vi "ex_InitTreeControl.vi"(4 "error in (no error)":errorcluster, 5 "File refnum in":refnum<k20>, 7 "reference":refnum<vi>) -> (0 "error out":errorcluster)   [LabVIEW 2017]
doc: "Initializes a Tree Control with the contents of the input file"
uses:
  <vilib>/Platform/storage/Storage.llb/Get Property (String).vi
  <vilib>/Platform/storage/Storage.llb/Get Property (Storage Refnums).vi
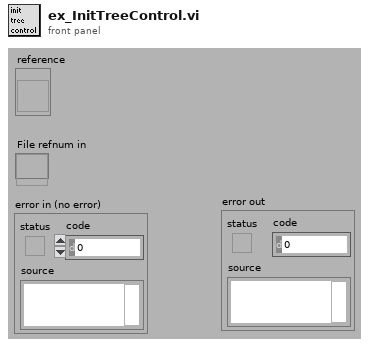
[diagram p1: front panel]
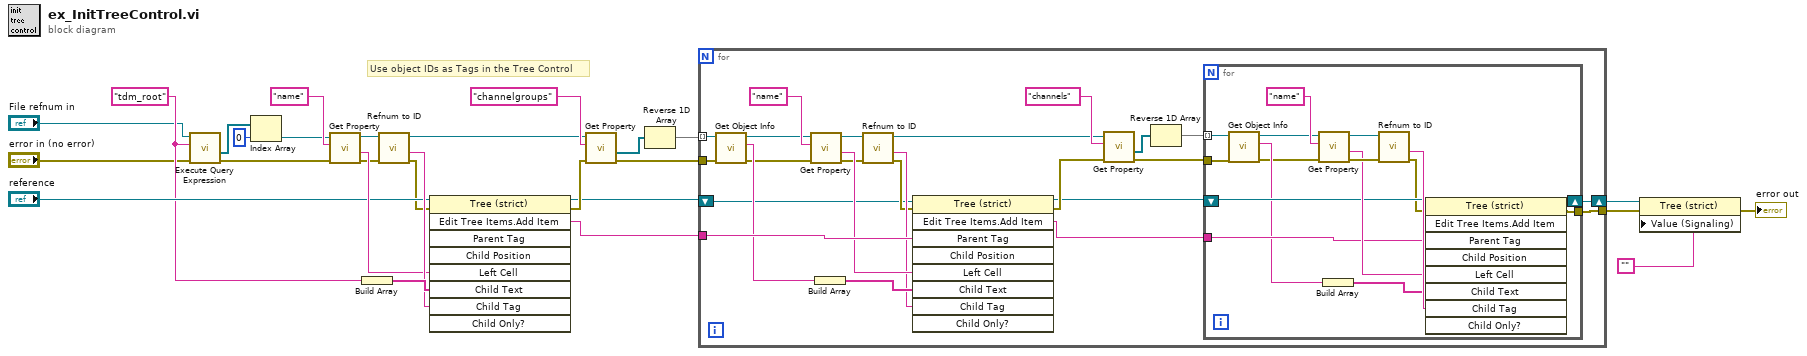
[diagram p0: block diagram]
diagram:
  w14 = "tdm_root" ("File")
  # "Use object IDs as Tags in the Tree Control"
  n1 = call <vilib>:"Execute Query Expression.vi"("error in (no error)"="error in (no error)", "object type"=w14, "storage refnum"="File refnum in") -> ("error out"=w16:errorcluster, "storage refnums"=w18:refnum<k20>[])  [unwired: 1 in, 2 out]
  n2 = Index Array(array=w18, index=0) -> (element=w19:refnum<k20>)
  n3 = call-poly <vilib>:"Get Property.vi"("error in (no error)"=w16, "Property name"="name" ("Name"), "storage refnum"=w19) -> ("error out"=w22:errorcluster, "Value"=w23:string, "storage refnum out"=w11:refnum<k20>)  [unwired: 6 out]
  n4 = Build Array(w14) -> (w25:string[])
  n5 = call <vilib>:"Refnum to ID.vi"("error in (no error)"=w22, "storage refnum"=w11) -> ("error out"=w10:errorcluster, "object ID"=w24:string, "storage refnum out"=w8:refnum<k20>)  [unwired: 3 out]
  n6 = invoke on="Invoke Node" class="Tree (strict)" method="Edit Tree Items.Add Item"(reference="reference", error in=w10, "Left Cell"=w23, "Child Text"=w25, "Child Tag"=w24) -> (reference out=w7:refnum<vi>, error out=w9:errorcluster, "Edit Tree Items:Add Item"=w27:string)  [unwired: 4 in, 6 out]
  n7 = call-poly <vilib>:"Get Property.vi"("error in (no error)"=w9, "Property name"="channelgroups" ("Channel groups"), "storage refnum"=w8) -> ("error out"=w26:errorcluster, "Value"=w1:refnum<k20>[])  [unwired: 7 out]
  n8 = Reverse 1D Array(array=w1) -> (reversed array=w2:refnum<k20>[])
  n9 = for {
    tunnel: w2 -> [w41] mode=indexing
    tunnel: w26 -> [w40]
    tunnel: w27 -> [w50]
    tunnel: [w42] -> w4
    shift-right: [w31] -> w6
    shift-left: w7 -> [w30]
    n10 = call <vilib>:"Get Object Info.vi"("error in (no error)"=w40, "storage refnum"=w41) -> ("error out"=w38:errorcluster, "object type"=w39:string, "storage refnum out"=w37:refnum<k20>)  [unwired: 7 out]
    n11 = call-poly <vilib>:"Get Property.vi"("error in (no error)"=w38, "Property name"="name" ("Name"), "storage refnum"=w37) -> ("error out"=w47:errorcluster, "Value"=w49:string, "storage refnum out"=w36:refnum<k20>)  [unwired: 6 out]
    n12 = Build Array(w39) -> (w48:string[])
    n13 = call <vilib>:"Refnum to ID.vi"("error in (no error)"=w47, "storage refnum"=w36) -> ("error out"=w34:errorcluster, "object ID"=w46:string, "storage refnum out"=w35:refnum<k20>)  [unwired: 3 out]
    n14 = invoke on="Invoke Node" class="Tree (strict)" method="Edit Tree Items.Add Item"(reference=w30, error in=w34, "Parent Tag"=w50, "Left Cell"=w49, "Child Text"=w48, "Child Tag"=w46) -> (reference out=w32:refnum<vi>, error out=w33:errorcluster, "Edit Tree Items:Add Item"=w45:string)  [unwired: 3 in, 6 out]
    n15 = call-poly <vilib>:"Get Property.vi"("error in (no error)"=w33, "Property name"="channels" ("Channels"), "storage refnum"=w35) -> ("error out"=w43:errorcluster, "Value"=w29:refnum<k20>[])  [unwired: 7 out]
    n16 = Reverse 1D Array(array=w29) -> (reversed array=w28:refnum<k20>[])
    n17 = for {
      tunnel: w43 -> [w57]
      tunnel: w45 -> [w61]
      tunnel: [w58] -> w42
      shift-right: [w53] -> w31
      shift-left: w32 -> [w60]
      tunnel: w28 -> [w52] mode=indexing
      n18 = call <vilib>:"Get Object Info.vi"("error in (no error)"=w57, "storage refnum"=w52) -> ("error out"=w54:errorcluster, "object type"=w56:string, "storage refnum out"=w55:refnum<k20>)  [unwired: 7 out]
      n19 = call-poly <vilib>:"Get Property.vi"("error in (no error)"=w54, "Property name"="name" ("Name"), "storage refnum"=w55) -> ("error out"=w65:errorcluster, "Value"=w63:string, "storage refnum out"=w66:refnum<k20>)  [unwired: 6 out]
      n20 = Build Array(w56) -> (w64:string[])
      n21 = call <vilib>:"Refnum to ID.vi"("error in (no error)"=w65, "storage refnum"=w66) -> ("error out"=w59:errorcluster, "object ID"=w67:string)  [unwired: 4 out]
      n22 = invoke on="Invoke Node" class="Tree (strict)" method="Edit Tree Items.Add Item"(reference=w60, error in=w59, "Parent Tag"=w61, "Left Cell"=w63, "Child Text"=w64, "Child Tag"=w67) -> (reference out=w53:refnum<vi>, error out=w58:errorcluster)  [unwired: 3 in, 7 out]
    }
  }
  n23 = property class="Tree (strict)"(reference=w6, error in=w4, "Value (Signaling)"="") -> (error out=→"error out":errorcluster)  [unwired: 1 out]
